vi "Request Notifications.vi"(6 "Return Priority (Normal)":T1=enum."Normal", 7 "Notification Msg (Type)":refnum<class "Notification Msg.lvclass">, 8 "error in (no error)":errorcluster, 9 "Data Type":variant, 10 "Topic Name":string, 11 "IObserver in":refnum<class "IObserver.lvclass">) -> (0 "error out":errorcluster, 3 "IObserver out":refnum<class "IObserver.lvclass">)   [LabVIEW 2015, in "IObserver.lvlib" / "IObserver.lvclass"]
uses:
  IObserver.lvclass
  Mediator/Transport Messages/Notification Msg/Notification Msg.lvclass
  <vilib>/ActorFramework/Message Enqueuer/Message Priority.ctl
  <vilib>/ActorFramework/Actor/Actor.lvclass/Actor.ctl
  <vilib>/ActorFramework/Message Enqueuer/Message Enqueuer.lvclass/Message Enqueuer.ctl
  IObserver Messages/Subscribe Msg/Subscribe Msg.lvclass/Subscribe Msg.ctl
  <vilib>/ActorFramework/Message Enqueuer/Init from Existing Queue.vi
  <vilib>/ActorFramework/Message Enqueuer/Enqueue.vi
  <vilib>/ActorFramework/Message Priority Queue/Priority Enqueue.vi
  <vilib>/ActorFramework/Message Enqueuer/Message Enqueuer.lvclass
  IObserver Messages/Subscribe Msg/Subscribe Msg.lvclass
  IMediator/SubscriptionRequest/SubscriptionRequest.lvclass
  <vilib>/ActorFramework/Actor/Actor.lvclass
  Mediator/Transport/ActorMessage/ActorMessage.lvclass
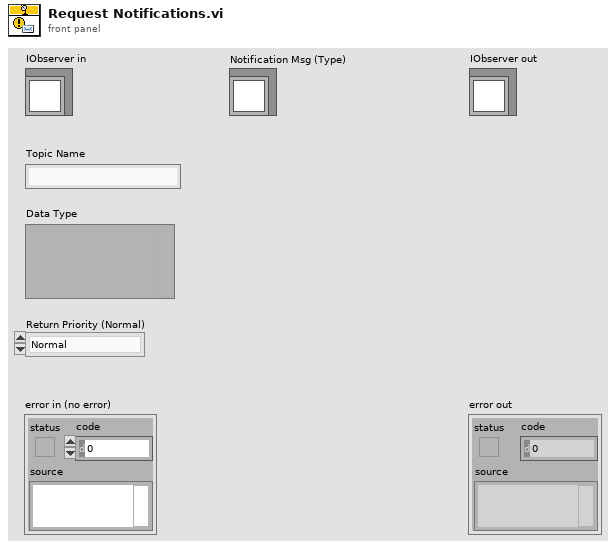
[diagram p1: front panel]
types:
  T1 = typedef "Actor Framework.lvlib/Message Enqueuer.lvclass/Message Priority.ctl" = enum16{"Low", "Normal", "High"}
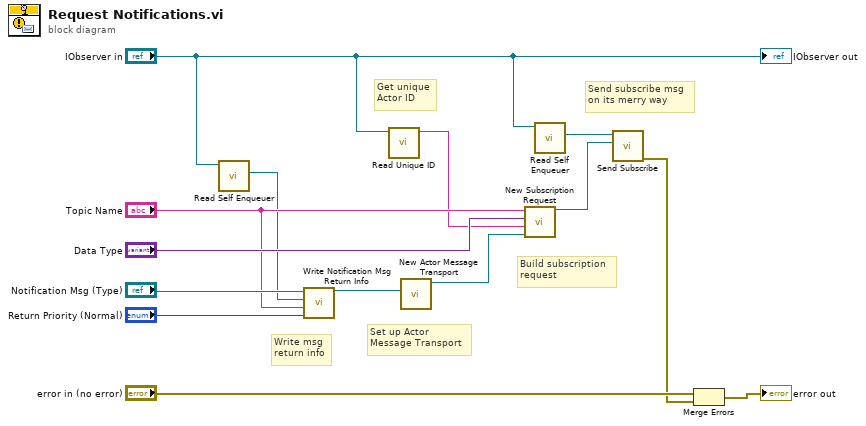
[diagram p0: block diagram]
diagram:
  # "Write msg\nreturn info"
  # "Send subscribe msg\non its merry way"
  # "Build subscription\nrequest"
  # "Get unique\nActor ID"
  # "Set up Actor\nMessage Transport"
  n1 = call <vilib>:"Read Self Enqueuer.vi"("Actor"="IObserver in") -> ("Self Enqueuer"=w2:refnum<class "Message Enqueuer.lvclass">)  [unwired: 10 in]
  n2 = call "Write Notification Msg Return Info.vi"("Return Priority (Normal)"="Return Priority (Normal)", "Topic Name"="Topic Name", "Message Enqueuer in"=w2, "Notification Msg"="Notification Msg (Type)") -> ("Notification Msg Out"=w8:refnum<class "Notification Msg.lvclass">)  [unwired: 7 in]
  n3 = call "Read Unique ID.vi"("IObserver In"="IObserver in") -> ("Unique ID"=w1:string)  [unwired: 10 in]
  n4 = call "New Actor Message Transport.vi"("Desired Notification Msg"=w8) -> ("ActorMessage out"=w13:refnum<class "ActorMessage.lvclass">)  [unwired: 9 in, 1 out]
  n5 = call "New Subscription Request.vi"("Transport"=w13, "Unique Subscriber ID"=w1, "Type"="Data Type", "Topic Name"="Topic Name") -> ("SubscriptionRequest out"=w11:refnum<class "SubscriptionRequest.lvclass">)  [unwired: 7 in]
  n6 = call <vilib>:"Read Self Enqueuer.vi"("Actor"="IObserver in") -> ("Self Enqueuer"=w12:refnum<class "Message Enqueuer.lvclass">)  [unwired: 10 in]
  n7 = call "Send Subscribe.vi"("SubscriptionRequest"=w11, "Message Enqueuer"=w12) -> ("error out"=w9:errorcluster)  [unwired: 8 in, 1 out]
  n8 = Merge Errors("error in (no error)", w9) -> (→"error out":errorcluster)
  "IObserver out" <- "IObserver in"
